vi "test-DC-Motor-Sim-Test2.vi"() -> (3 "All Passed":bool)   [LabVIEW 2019]
uses:
  <vilib>/Rock Robotics/WPI/ThirdParty/JAS_Junk/TrajLib/DCMOTOR_TYPES_ENUM.ctl
  <vilib>/Analysis/Matrix/Datatypes/RealMatrix.ctl
  <vilib>/Rock Robotics/WPI/ThirdParty/JAS_Junk/TrajLib/DCMotor_GetCIM.vi
  <vilib>/Rock Robotics/WPI/ThirdParty/JAS_Junk/TrajLib/DCMotor_GetAndymark9015.vi
  <vilib>/Rock Robotics/WPI/ThirdParty/JAS_Junk/TrajLib/DCMotor_GetAndymarkRs775_125.vi
  <vilib>/Rock Robotics/WPI/ThirdParty/JAS_Junk/TrajLib/DCMotor_GetBag.vi
  <vilib>/Rock Robotics/WPI/ThirdParty/JAS_Junk/TrajLib/DCMotor_GetBanebotsRs550.vi
  <vilib>/Rock Robotics/WPI/ThirdParty/JAS_Junk/TrajLib/DCMotor_GetBanebotsRs775.vi
  <vilib>/Rock Robotics/WPI/ThirdParty/JAS_Junk/TrajLib/DCMotor_GetFalcon500.vi
  <vilib>/Rock Robotics/WPI/ThirdParty/JAS_Junk/TrajLib/DCMotor_GetMiniCIM.vi
  <vilib>/Rock Robotics/WPI/ThirdParty/JAS_Junk/TrajLib/DCMotor_GetNEO.vi
  <vilib>/Rock Robotics/WPI/ThirdParty/JAS_Junk/TrajLib/DCMotor_GetNEO550.vi
  <vilib>/Rock Robotics/WPI/ThirdParty/JAS_Junk/TrajLib/DCMotor_GetRomiBuiltIn.vi
  <vilib>/Rock Robotics/WPI/ThirdParty/JAS_Junk/TrajLib/DCMotor_GetVex775Pro.vi
  <vilib>/Rock Robotics/WPI/ThirdParty/JAS_Junk/TrajLib/PIDController_Calculate_SP_PV.vi
  <vilib>/Rock Robotics/WPI/ThirdParty/JAS_Junk/TrajLib/PIDController_AtSetpoint.vi
  <vilib>/Rock Robotics/WPI/ThirdParty/JAS_Junk/TrajLib/PIDController_SetPID.vi
  <vilib>/Rock Robotics/WPI/ThirdParty/JAS_Junk/TrajLib/PIDController_SetIntegratorRange.vi
  <vilib>/Rock Robotics/WPI/ThirdParty/JAS_Junk/TrajLib/PIDController_SetTolerancePandV.vi
  <vilib>/Rock Robotics/WPI/ThirdParty/JAS_Junk/TrajLib/PIDController_DisableContinousInput.vi
  <vilib>/Rock Robotics/WPI/ThirdParty/JAS_Junk/TrajLib/PIDController_EnableContinousInput.vi
  <vilib>/Rock Robotics/WPI/ThirdParty/JAS_Junk/TrajLib/PIDController_Reset.vi
  <vilib>/Rock Robotics/WPI/ThirdParty/JAS_Junk/TrajLib/PIDController_NewPeriod.vi
  <vilib>/Rock Robotics/WPI/ThirdParty/JAS_Junk/TrajLib/BatterySim_CalculateLoadedBatteryVoltage.vi
  <vilib>/Rock Robotics/WPI/ThirdParty/JAS_Junk/TrajLib/DCMotor_New.vi
  <vilib>/Rock Robotics/WPI/ThirdParty/JAS_Junk/TrajLib/Units_RotationsPerMinuteToRadiansPerSecond.vi
  <vilib>/Rock Robotics/WPI/ThirdParty/JAS_Junk/TrajLib/PIDController_SetSetpoint.vi
  <vilib>/Rock Robotics/WPI/ThirdParty/JAS_Junk/TrajLib/PIDController_Calculate_PV.vi
  <vilib>/Rock Robotics/WPI/ThirdParty/JAS_Junk/TrajLib/ControllerUtil_GetModulusError.vi
  <vilib>/Rock Robotics/SystemInterfaces/NetworkCommunication/NetComm_UsageReport_report.vi
  <vilib>/Rock Robotics/WPI/ThirdParty/JAS_Junk/TrajLib/Util_LibraryGlobals.vi
  <vilib>/Rock Robotics/WPI/ThirdParty/JAS_Junk/TrajLib/Trajectory_Library.lvlib
  <vilib>/Analysis/Matrix/NI_Matrix.lvlib
panel:
  out "Pos Control Passed":bool
  out "Pos Ctrl":T1(graph)
  out "Error":bool
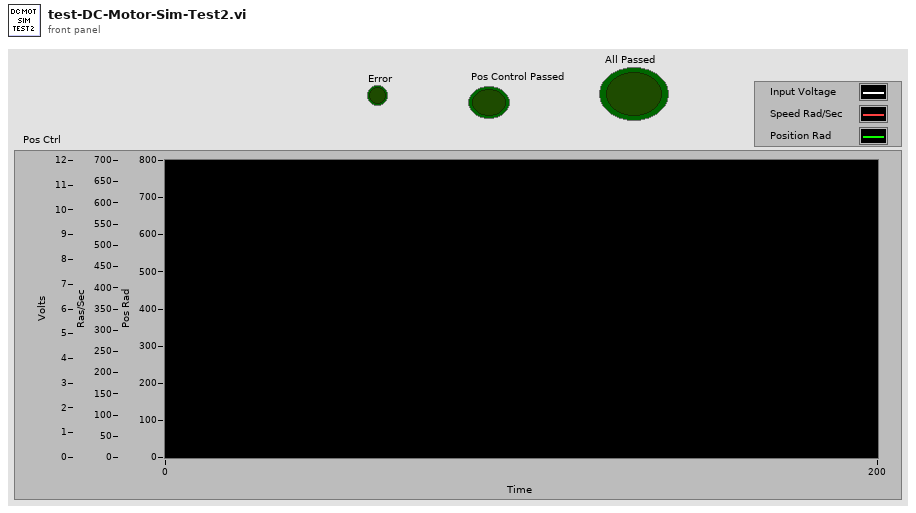
[diagram p1: front panel]
types:
  T1 = cluster{dbl, "Velocity_RadPerSec":dbl, "Position_Rad":dbl}
  T2 = typedef "NI_Matrix.lvlib/RealMatrix.ctl" = dbl[][]
  T3 = typedef "Trajectory_Library.lvlib/DCMOTOR_TYPES_ENUM.ctl" = enum16{"CIM", "AndyMark 9015", "Andy Mark RS 775 125", "Bag", "BaneBots RS 550", "BaneBots RS 775", "Falcon 500", "Mini CIM", "NEO", "NEO 550", "Romi BuiltIn", "Vex 775 Pro"}
  T4 = typedef "Trajectory_Library.lvlib/DCMOTOR.CTL" = cluster{"nominalVoltage_Volts":dbl, "StallTorque_NM":dbl, "StallCurrent_Amps":dbl, "FreeCurrent_Amps":dbl, "FreeSpeed_RadPerSec":dbl, "R_Ohms":dbl, "KvINV_RadPerSecPerVolt":dbl, "Kt_NMPerAmp":dbl, "L_H":dbl, "Jr_KgM2":dbl}
  T5 = typedef "Trajectory_Library.lvlib/DCMOTOR_SIM.ctl" = cluster{"LinearSystemSim":T6, "GearBox":T4, "Gearing":dbl}
  T6 = typedef "Trajectory_Library.lvlib/LINEAR_SYSTEM_SIM.ctl" = cluster{"m_Plant":T7, "m_X":T2, "m_Y":T2, "m_U":T2, "MeasureStdDev":T2}
  T7 = typedef "Trajectory_Library.lvlib/LINEAR_SYSTEM.ctl" = cluster{"m_A":T2, "m_B":T2, "m_C":T2, "m_D":T2, "States":i32, "Inputs":i32, "Outputs":i32}
  T8 = typedef "Trajectory_Library.lvlib/PID_TUNING.ctl" = cluster{"Kp":dbl, "Ki":dbl, "Kd":dbl, "MaximumIntegral":dbl, "MinimumIntegral":dbl}
  T9 = typedef "Trajectory_Library.lvlib/PID_INPUT_LIMITS.ctl" = cluster{"MaxInput":dbl, "MinInput":dbl, "Continuous":bool}
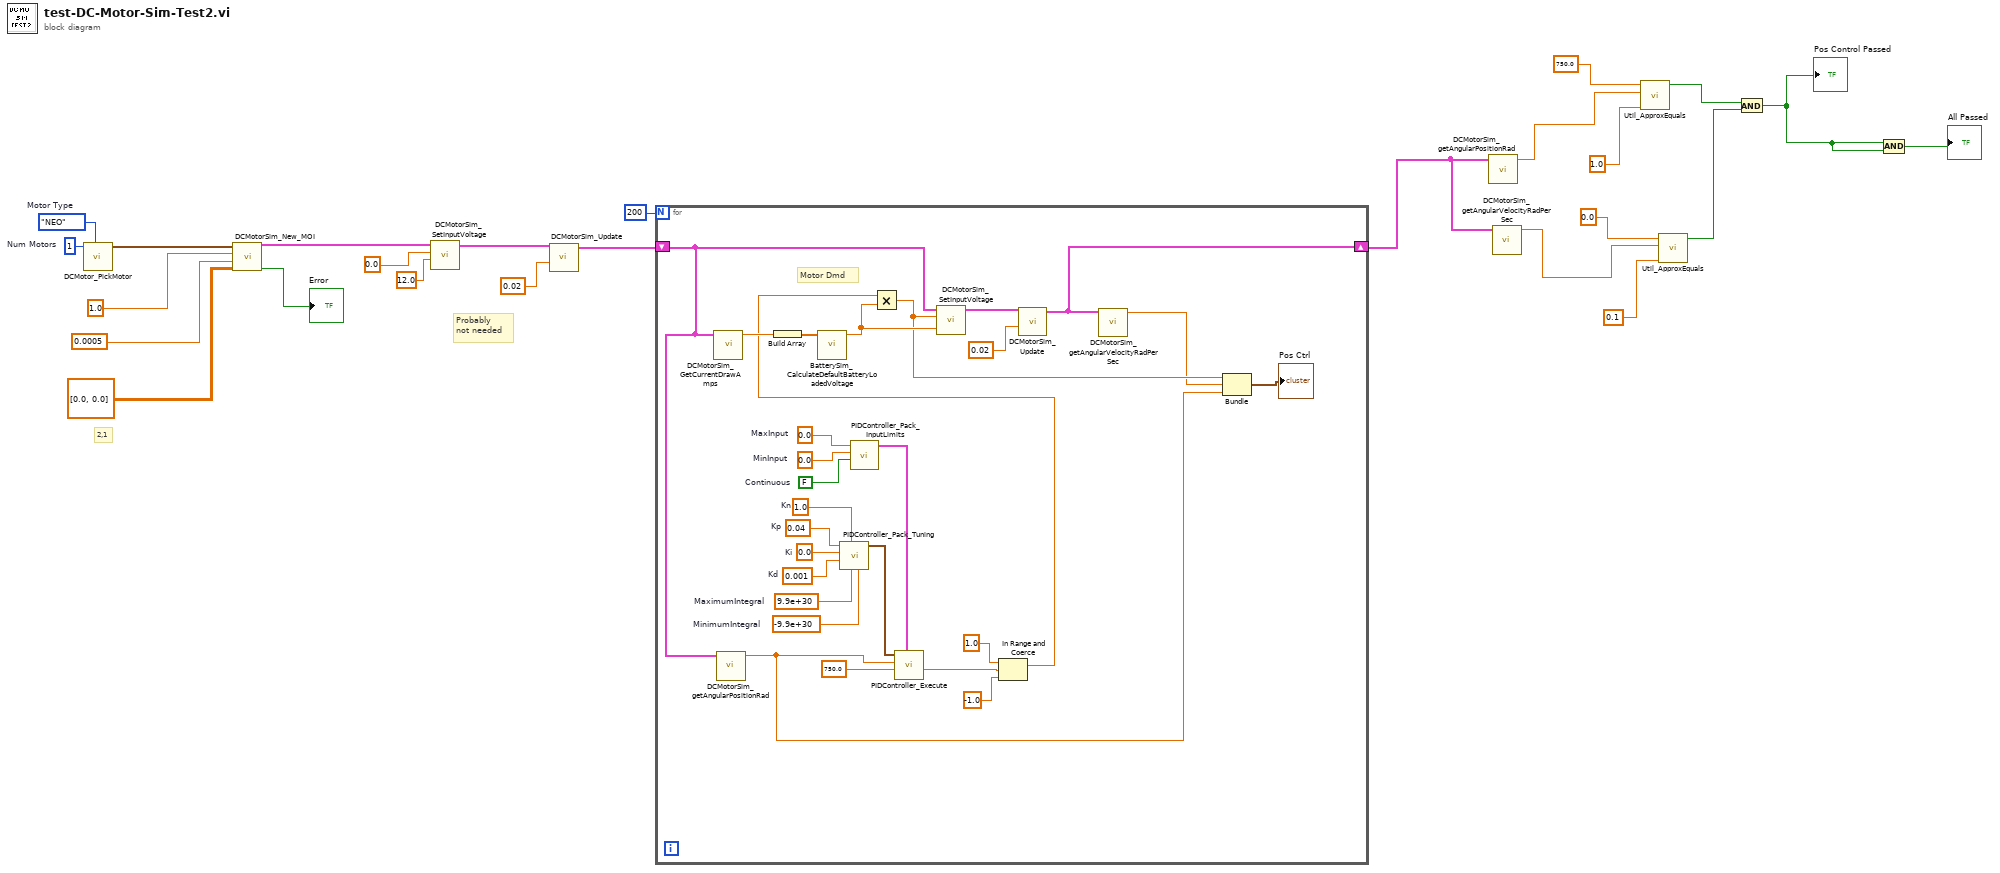
[diagram p0: block diagram]
diagram:
  w25 = 1  # Num Motors
  w24 = DCMOTOR_TYPES_ENUM."NEO"  # Motor Type
  # "Probably \nnot needed"
  # "2,1"
  n1 = call <vilib>:"DCMotor_PickMotor.vi"("DCMOTOR_TYPES"=w24, "Num Motors"=w25) -> ("DCMOTOR"=w12:T4)  [unwired: 9 in]
  n2 = call <vilib>:"DCMotorSim_New_MOI.vi"("MeasurementStdDev"=T2 [[0.0], [0.0]], "jKgMetersSquared"=0.0005, "Gearing"=1.0, "GearBox"=w12) -> ("Error"=→"Error":bool, "DCMotorSim"=w18:T5)  [unwired: 6 in]
  n3 = call <vilib>:"DCMotorSim_SetInputVoltage.vi"("Battery_Volts"=12.0, "Volts"=0.0, "DCMotorSim"=w18) -> ("out DCMotorSim"=w14:T5)  [unwired: 8 in]
  n4 = call <vilib>:"DCMotorSim_Update.vi"("dT_Seconds"=0.02, "DCMotorSim"=w14) -> ("out DCMotorSim"=w13:T5)  [unwired: 8 in, 1 out]
  n5 = for {
    N: 200 -> [_]
    shift-right: [w44] -> w7
    shift-left: w13 -> [w31]
    w43 = 1.0  # Kn
    w42 = 0.0  # MaxInput
    w41 = 0.0  # MinInput
    w40 = FALSE  # Continuous
    w39 = 0.04  # Kp
    w38 = 0.0  # Ki
    w37 = 0.001  # Kd
    w36 = 9.9e+30  # MaximumIntegral
    w35 = -9.9e+30  # MinimumIntegral
    # "Motor Dmd"
    n6 = call <vilib>:"DCMotorSim_GetCurrentDrawAmps.vi"("DCMotorSim"=w31) -> ("Current_Amps"=w51:dbl)  [unwired: 10 in]
    n7 = call <vilib>:"DCMotorSim_getAngularPositionRad.vi"("DCMotorSim"=w31) -> ("Position_Rad"=w26:dbl)  [unwired: 10 in]
    n8 = Build Array(w51) -> (w52:dbl[])
    n9 = call <vilib>:"BatterySim_CalculateDefaultBatteryLoadedVoltage.vi"("Currents"=w52) -> ("Voltage"=w50:dbl)  [unwired: 10 in]
    n10 = call <vilib>:"PIDController_Pack_Tuning.vi"("MinimumIntegral"=w35, "MaximumIntegral"=w36, "Kn"=w43, "Kd"=w37, "Ki"=w38, "Kp"=w39) -> ("PID Tuning"=w34:T8)  [unwired: 5 in]
    n11 = call <vilib>:"PIDController_Pack_InputLimits.vi"("Continuous"=w40, "MinInput"=w41, "MaxInput"=w42) -> ("PID Input Limits"=w33:T9)  [unwired: 8 in]
    n12 = call <vilib>:"PIDController_Execute.vi"("PID Input Limits"=w33, "SP-SetPoint"=750.0, "PV-Measurement"=w26, "PID Tuning"=w34) -> ("CO-ControlOutput"=w28:dbl)  [unwired: 5 in, 2 out]
    n13 = In Range and Coerce(upper limit=1.0, x=w28, lower limit=-1.0) -> (coerced(x)=w27:dbl)  [unwired: 1 out]
    n14 = Multiply(x=w27, y=w50) -> (x*y=w46:dbl)
    n15 = call <vilib>:"DCMotorSim_SetInputVoltage.vi"("Battery_Volts"=w50, "Volts"=w46, "DCMotorSim"=w31) -> ("out DCMotorSim"=w49:T5)  [unwired: 8 in]
    n16 = call <vilib>:"DCMotorSim_Update.vi"("dT_Seconds"=0.02, "DCMotorSim"=w49) -> ("out DCMotorSim"=w44:T5)  [unwired: 8 in, 1 out]
    n17 = call <vilib>:"DCMotorSim_getAngularVelocityRadPerSec.vi"("DCMotorSim"=w44) -> ("Velocity_RadPerSec"=w45:dbl)  [unwired: 10 in]
    n18 = Bundle(w46, "Velocity_RadPerSec"=w45, "Position_Rad"=w26) -> (→"Pos Ctrl":T1)  [unwired: 1 in]
  }
  n19 = call <vilib>:"DCMotorSim_getAngularPositionRad.vi"("DCMotorSim"=w7) -> ("Position_Rad"=w8:dbl)  [unwired: 10 in]
  n20 = call <vilib>:"DCMotorSim_getAngularVelocityRadPerSec.vi"("DCMotorSim"=w7) -> ("Velocity_RadPerSec"=w4:dbl)  [unwired: 10 in]
  n21 = call <vilib>:"Util_ApproxEquals.vi"("Tolerance"=1.0, "Value 2"=w8, "Value 1"=750.0 ("y")) -> ("ApproxEquals"=w3:bool)  [unwired: 8 in]
  n22 = call <vilib>:"Util_ApproxEquals.vi"("Tolerance"=0.1, "Value 2"=w4, "Value 1"=0.0 ("y")) -> ("ApproxEquals"=w2:bool)  [unwired: 8 in]
  n23 = And(x=w3, y=w2) -> (x .and. y?=w1:bool)
  "Pos Control Passed" <- w1
  n24 = And(x=w1, y=w1) -> (x .and. y?=→"All Passed":bool)
